vi "Check.vi"(1 "Queue in":refnum<queue>, 2 "Grids":i32[][](array[numeric])) -> (0 "Movable?":bool)   [LabVIEW 2018]
doc: "Check if the user won or losed."
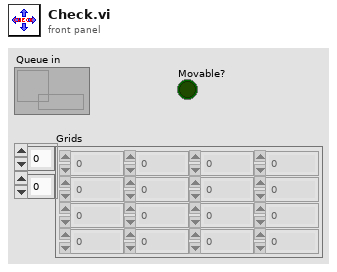
[diagram p1: front panel]
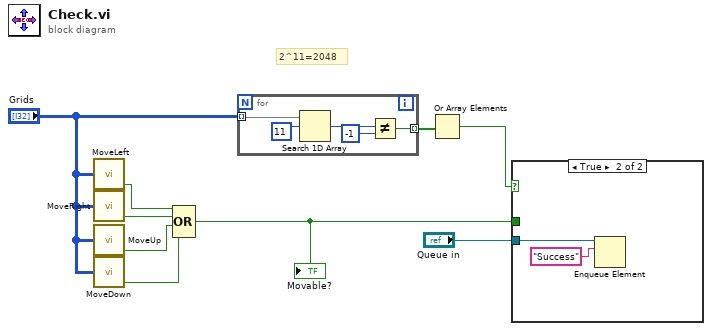
[diagram p0: block diagram]
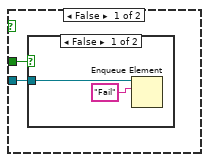
[diagram p2: hidden frame]
diagram:
  # "2^11=2048"
  n1 = call "MoveLeft.vi"("Grids In"="Grids") -> ("Moved?"=w1:bool)  [unwired: 2 out]
  n2 = call "MoveRight.vi"("Grids In"="Grids") -> ("Moved?"=w2:bool)  [unwired: 2 out]
  n3 = call "MoveUp.vi"("Grids In"="Grids") -> ("Moved?"=w3:bool)  [unwired: 2 out]
  n4 = call "MoveDown.vi"("Grids In"="Grids") -> ("Moved?"=w4:bool)  [unwired: 2 out]
  n5 = Compound Arithmetic op=OR(w1, w2, w3, w4) -> (w9:bool)
  "Movable?" <- w9
  n6 = for {
    tunnel: "Grids" -> [w14] mode=indexing
    tunnel: [w10] -> w6 mode=indexing
    n7 = Search 1D Array(1D array=w14, element=11) -> (index of element=w12:i32)  [unwired: 1 in]
    n8 = Not Equal?(x=w12, y=-1) -> (x != y?=w10:bool)
  }
  n9 = Or Array Elements(Boolean array=w6) -> (logical OR=w7:bool)
  n10 = case shown="True" w7 {
    tunnel: "Queue in" -> [w15 w20]
    tunnel: w9 -> [w16 _]
    frame False {
      n11 = case shown="False" w16 {
        tunnel: w15 -> [w18 _]
        frame False {
          n12 = Enqueue Element(queue=w18, element="Fail") -> ()  [unwired: 2 in, 3 out]
        }
        frame True {
        }
      }
    }
    frame True {
      n13 = Enqueue Element(queue=w20, element="Success") -> ()  [unwired: 2 in, 3 out]
    }
  }
